vi "tank control.vi"() -> ()   [LabVIEW 2016]
panel:
  out "?":dbl
  out "?":dbl
  out "?":dbl
  in  "Reset":bool
  in  "?":bool
  in  "?":bool
  out "Slide 3":dbl(slide) scale=0.0..100.0
  out "?":bool
  out "?":dbl(slide) scale=0.0..10.0
  out "Slide":u8(slide) scale=0.0..10.0
  # "start"
  # "stop"
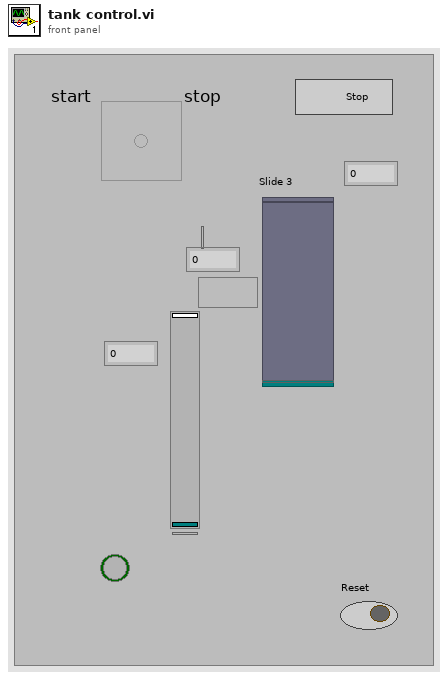
[diagram p1: front panel]
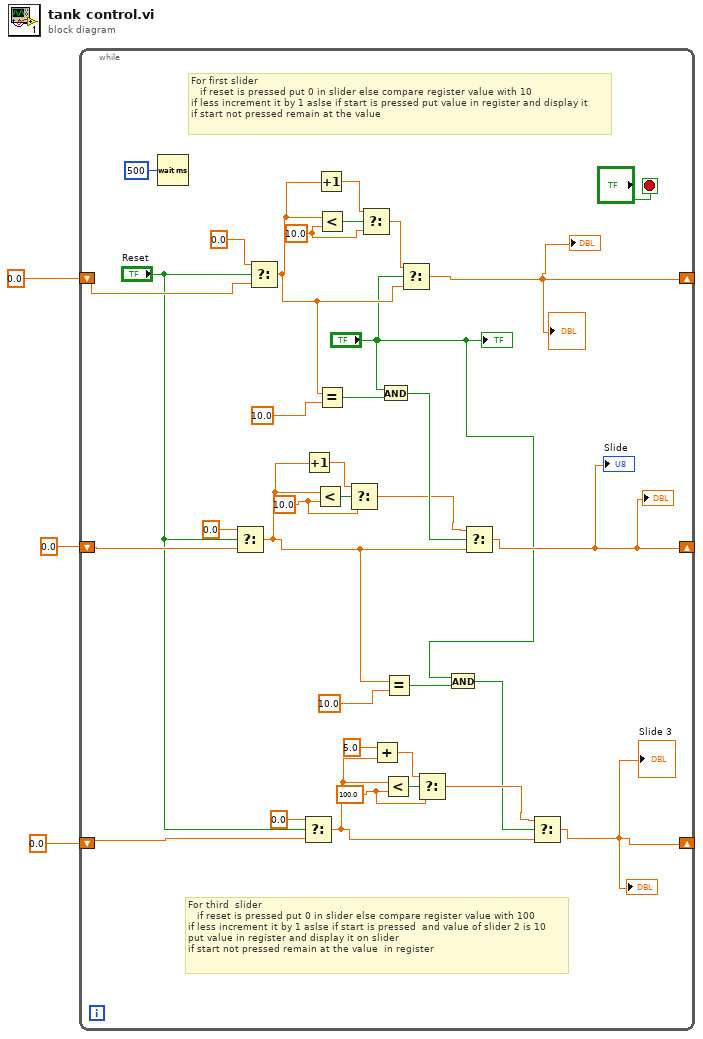
[diagram p0: block diagram]
diagram:
  n1 = while {
    shift-right: [w35] -> _
    shift-left: 0.0 -> [w26]
    shift-right: [w19] -> _
    shift-left: 0.0 ("f") -> [w30]
    shift-right: [w6] -> _
    shift-left: 0.0 ("f") -> [w12]
    stop <- "?" stop-if-true
    w16 = 100.0 ("y")
    w22 = 10.0 ("y")
    w32 = 10.0 ("y")
    # "For third  slider      \n   if reset is pressed put 0 in slider else compare register value with 100\nif less increment it by 1 aslse if start is pressed  and value of slider 2 is 10 \nput value in register and display it on slider\nif start not pressed remain at the value  in register"
    # "For first slider      \n   if reset is pressed put 0 in slider else compare register value with 10\nif less increment it by 1 aslse if start is pressed put value in register and display it\nif start not pressed remain at the value"
    n2 = Wait (ms)(milliseconds to wait=u32 500) -> ()  [unwired: 1 out]
    n3 = Select(t=0.0, s="Reset", f=w30) -> (s? t:f=w7:dbl)
    n4 = Select(t=0.0, s="Reset", f=w26) -> (s? t:f=w24:dbl)
    n5 = Select(t=0.0, s="Reset", f=w12) -> (s? t:f=w5:dbl)
    n6 = Increment(x=w7) -> (x+1=w21:dbl)
    n7 = Less?(x=w7, y=w22) -> (x < y?=w23:bool)
    n8 = Increment(x=w24) -> (x+1=w33:dbl)
    n9 = Less?(x=w24, y=w32) -> (x < y?=w34:bool)
    n10 = Equal?(x=w24, y=10.0) -> (x = y?=w28:bool)
    n11 = Select(t=w21, s=w23, f=w22) -> (s? t:f=w20:dbl)
    n12 = Select(t=w33, s=w34, f=w32) -> (s? t:f=w31:dbl)
    n13 = Add(x=5.0, y=w5) -> (x+y=w15:dbl)
    n14 = And(x="?", y=w28) -> (x .and. y?=w25:bool)
    n15 = Less?(x=w5, y=w16) -> (x < y?=w17:bool)
    n16 = Equal?(x=w7, y=10.0) -> (x = y?=w11:bool)
    n17 = Select(t=w31, s="?", f=w24) -> (s? t:f=w35:dbl)
    "?" <- w35
    "?" <- w35
    n18 = Select(t=w15, s=w17, f=w16) -> (s? t:f=w14:dbl)
    n19 = And(x="?", y=w11) -> (x .and. y?=w9:bool)
    n20 = Select(t=w20, s=w25, f=w7) -> (s? t:f=w19:dbl)
    "Slide" <- w19
    "?" <- w19
    n21 = Select(t=w14, s=w9, f=w5) -> (s? t:f=w6:dbl)
    "Slide 3" <- w6
    "?" <- w6
    "?" <- "?"
  }
